vi "Read Circle Radius.vi"   [LabVIEW 2011, in "LVH-Leap.lvlib"]
uses:
  LVH-Leap.lvlib
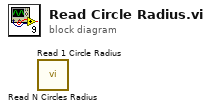
[diagram p0: block diagram]
diagram:
  n1 = call "Read N Circles Radius.vi"() -> ()  [unwired: 8 in, 4 out]
  n2 = call "Read 1 Circle Radius.vi"() -> ()  [unwired: 8 in, 4 out]
